vi "Stop Core.vi"(10 "final error code":i32, 11 "Event Source In":refnum<class "Event Source Actor.lvclass">) -> (3 "Event Source Out":refnum<class "Event Source Actor.lvclass">)   [LabVIEW 2021, in "EventSourceActor.lvlib" / "Event Source.lvlib" / "Event Source Actor.lvclass"]
doc: "(<B>Filename</B>: Actor Framework.lvlib:Actor.lvclass:Stop Core.vi)\n\nDefines what the actor does before it stops. Use the <B>final error code</B> input to determine whether the actor shut down in response to an error.\n\nBy default, this method does nothing. A descendant class may override it to define behavior, such as shutting down any processes the actor initiated in its override of the Actor Core method."
uses:
  Event Source Actor.lvclass
  Event Source Actor.lvclass/Event Source Actor.ctl
  <vilib>/ActorFramework/Actor/Actor.lvclass
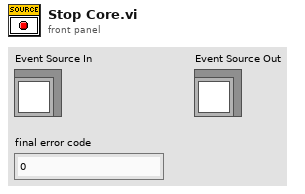
[diagram p1: front panel]
types:
  T1 = map{string, set{refnum<class "Message Enqueuer.lvclass">}}
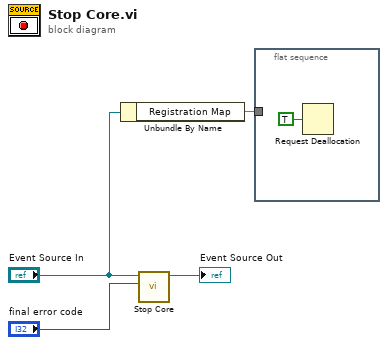
[diagram p0: block diagram]
diagram:
  n1 = Unbundle By Name("Event Source In") -> ("Registration Map"=w1:T1)
  n2 = call-parent "Stop Core.vi"("final error code"="final error code", "Actor in"="Event Source In") -> ("Actor out"=→"Event Source Out":refnum<class "Event Source Actor.lvclass">)  [unwired: 9 in]
  n3 = flat-sequence {
    tunnel: w1 -> [_]
    frame #0 {
      n4 = Request Deallocation(TRUE ("flag")) -> ()
    }
  }
